vi "FVIR_LDO_Agilent_DisplayString.vi"(11 "Agilent Data in":T1) -> (3 "transposed array":string[][](array[string]))   [LabVIEW 2020]
uses:
  Agilent Data.ctl
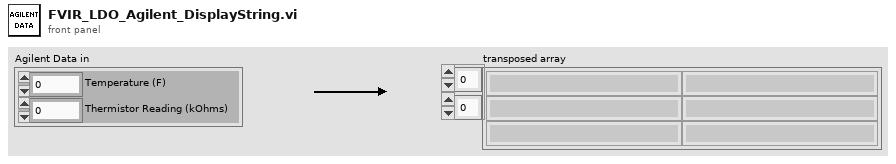
[diagram p1: front panel]
types:
  T1 = typedef "Agilent Data.ctl" = cluster{"Temperature (F)":dbl, "Thermistor Reading (kOhms)":dbl}
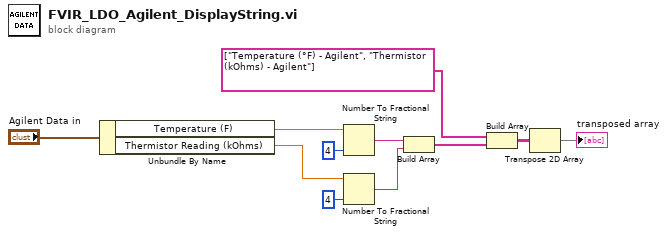
[diagram p0: block diagram]
diagram:
  n1 = Unbundle By Name("Agilent Data in") -> ("Temperature (F)"=w10:dbl, "Thermistor Reading (kOhms)"=w9:dbl)
  n2 = Number To Fractional String(number=w10, precision (6)=i16 4) -> (F-format string=w6:string)  [unwired: 2 in]
  n3 = Number To Fractional String(number=w9, precision (6)=i16 4) -> (F-format string=w5:string)  [unwired: 2 in]
  n4 = Build Array(w6, w5) -> (w3:string[])
  n5 = Build Array(string[] ["Temperature (°F) - Agilent", "Thermistor (kOhms) - Agilent"], w3) -> (w2:string[][])
  n6 = Transpose 2D Array(2D array=w2) -> (transposed array=→"transposed array":string[][])
